vi "SVN directory.vi"(6 "Ini":T1, 8 "error in (no error)":errorcluster, 11 "Sourceforge Directory in":bool) -> (0 "error out":errorcluster, 3 "Sourceforge Directory out":bool)   [LabVIEW 2010]
uses:
  ini control.ctl
  <vilib>/Utility/config.llb/Read Key (Boolean).vi
  <vilib>/Utility/config.llb/Write Key (Boolean).vi
  <vilib>/Utility/config.llb/NI_LVConfig.lvlib
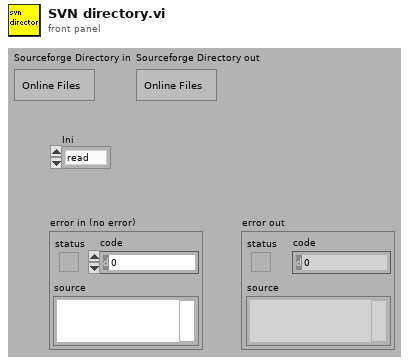
[diagram p1: front panel]
types:
  T1 = typedef "ini control.ctl" = enum16{"read", "write"}
  T2 = typedef "NI_LVConfig.lvlib/Config Data RefNum.ctl" = refnum<k1>
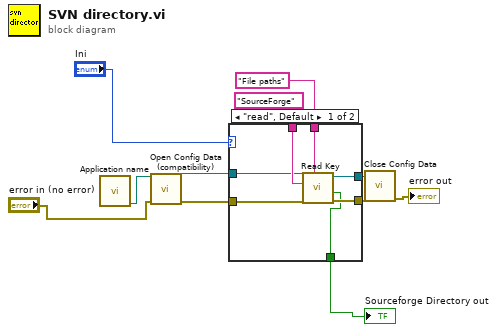
[diagram p0: block diagram]
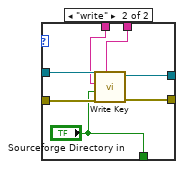
[diagram p2: hidden frame]
diagram:
  n1 = call "Application name.vi"() -> ("Ini file path"=w7:path)  [unwired: 4 in, 3 out]
  n2 = call <vilib>:"Open Config Data (compatibility).vi"("error in (no error)"="error in (no error)", "configuration file path"=w7) -> ("error out"=w9:errorcluster, "refnum"=w10:T2)  [unwired: 7 in, 1 out]
  n3 = case shown="\"read\", Default" "Ini" {
    tunnel: "SourceForge" ("key") -> [w18 w23]
    tunnel: w10 -> [w17 w24]
    tunnel: w9 -> [w16 w25]
    tunnel: "File paths" ("section") -> [w15 w22]
    tunnel: [w14 w20] -> w5
    tunnel: [w13 w21] -> w4
    tunnel: [w12 "Sourceforge Directory in"] -> w1
    frame "read", Default {
      n4 = call-poly <vilib>:"Read Key.vi"("section"=w15, "error in (no error)"=w16, "key"=w18, "refnum"=w17) -> ("error out"=w14:errorcluster, "value"=w12:bool, "refnum out"=w13:T2)  [unwired: 4 in, 1 out]
    }
    frame "write" {
      n5 = call-poly <vilib>:"Write Key.vi"("section"=w22, "error in (no error)"=w25, "value"="Sourceforge Directory in", "key"=w23, "refnum"=w24) -> ("error out"=w20:errorcluster, "refnum out"=w21:T2)  [unwired: 4 in, 1 out]
    }
  }
  "Sourceforge Directory out" <- w1
  n6 = call <vilib>:"Close Config Data.vi"("error in (no error)"=w5, "refnum"=w4) -> ("error out"=→"error out":errorcluster)  [unwired: 8 in, 1 out]
